vi "Lift Joystick Activity.vi"(11 "Operator Gamepad":T1) -> (1 "Active?":bool, 2 "Axes":dbl[](array[numeric]), 3 "Gamepad Out":T1)   [LabVIEW 2014]
uses:
  <vilib>/Rock Robotics/WPI/Joystick/WPI_JoystickDevRef.ctl
  <vilib>/Rock Robotics/WPI/Joystick/WPI_JoystickDeviceEnum.ctl
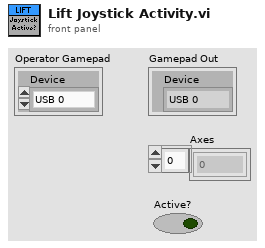
[diagram p1: front panel]
types:
  T1 = typedef "WPI_JoystickDevRef.ctl" = cluster{"Device":T2}
  T2 = typedef "WPI_JoystickDeviceEnum.ctl" = enum16{"USB 0", "USB 1", "USB 2", "USB 3", "USB 4", "USB 5"}
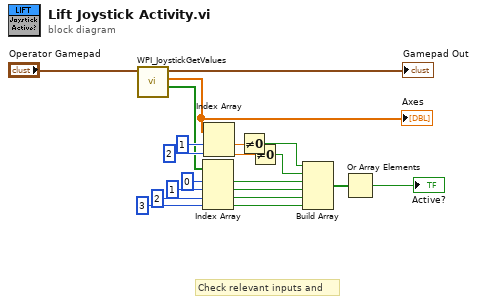
[diagram p0: block diagram]
diagram:
  # "Check relevant inputs and"
  n1 = call <vilib>:"WPI_JoystickGetValues.vi"("JoystickDevRef"="Operator Gamepad") -> ("Buttons"=w3:bool[], "Axes"=w8:dbl[], "JoystickDevRef"=→"Gamepad Out":T1)  [unwired: 6 in, 2 out]
  "Axes" <- w8
  n2 = Index Array(array=w3, index #1=0 ("index"), index #2=1 ("index"), index #3=2 ("index"), index #4=3 ("index")) -> (element #1=w15:bool, element #2=w16:bool, element #3=w17:bool, element #4=w18:bool)
  n3 = Index Array(array=w8, index #1=1 ("index"), index #2=2 ("index")) -> (element #1=w11:dbl, element #2=w12:dbl)
  n4 = Not Equal To 0?(x=w11) -> (x != 0?=w13:bool)
  n5 = Not Equal To 0?(x=w12) -> (x != 0?=w14:bool)
  n6 = Build Array(w13, w14, w15, w16, w17, w18) -> (w19:bool[])
  n7 = Or Array Elements(Boolean array=w19) -> (logical OR=→"Active?":bool)
